vi "Read_camFrameRate.vi"() -> (3 "cam_FrameRate":sgl)   [LabVIEW 2023, in "Cam Data.lvlib"]
uses:
  Cam Data.lvlib
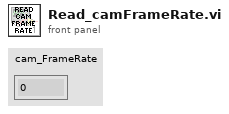
[diagram p1: front panel]
types:
  T1 = cluster{"Address IP":string, "Rack":i32, "Slot ":i32, "DB Number":i32, "Start":i32, "Amount":i32}
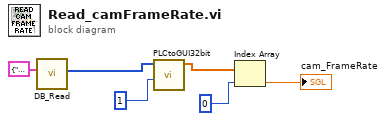
[diagram p0: block diagram]
diagram:
  n1 = call "DB_Read.vi"("Input Params"=T1 {"Address IP"="192.168.10.80", "Rack"=0, "Slot "=2, "DB Number"=18, "Start"=56, "Amount"=4}) -> ("Data"=w5:u8[])  [unwired: 8 in, 2 out]
  n2 = call "PLCtoGUI32bit.vi"("DB Val Qty"=u16 1, "DB Input Vals"=w5) -> ("RealValue"=w3:sgl[])  [unwired: 9 in]
  n3 = Index Array(array=w3, index=0) -> (element=→"cam_FrameRate":sgl)
